vi "记录转表格.vi"(2 "记录":T1(array[cluster])) -> (16 "表格":string[][](array[string]))   [LabVIEW 2019, in "MainPage.lvlib" / "MainPage.lvclass"]
uses:
  MainPage.lvclass
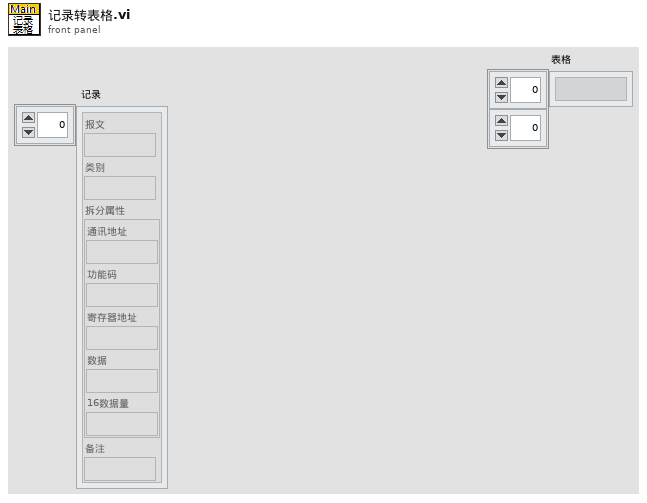
[diagram p1: front panel]
types:
  T1 = cluster{"报文":string, "类别":string, "拆分属性":cluster{"通讯地址":string, "功能码":string, "寄存器地址":string, "数据":string, "16数据量":string}, "备注":string}[]
  T2 = cluster{"报文":string, "类别":string, "拆分属性":cluster{"通讯地址":string, "功能码":string, "寄存器地址":string, "数据":string, "16数据量":string}, "备注":string}
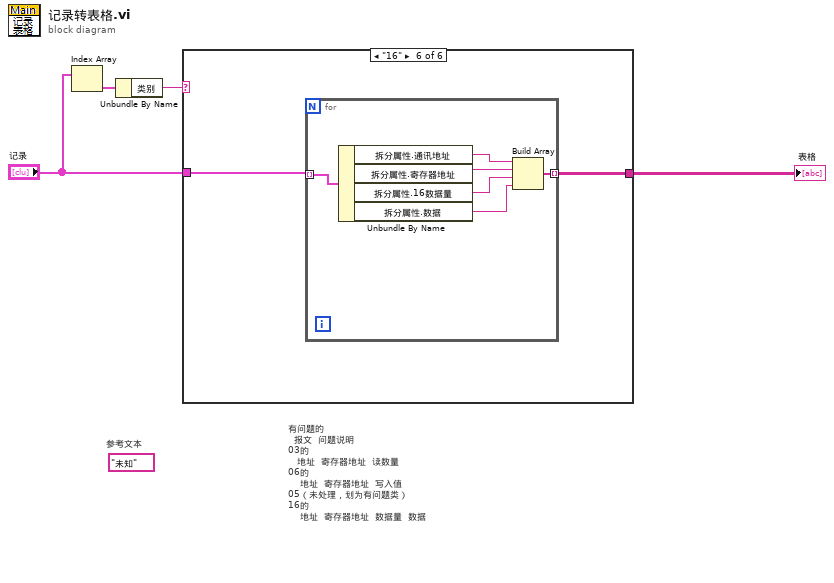
[diagram p0: block diagram]
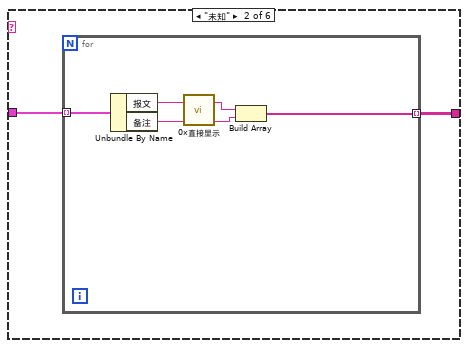
[diagram p3: hidden frame]
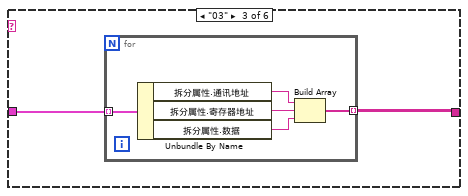
[diagram p4: hidden frame]
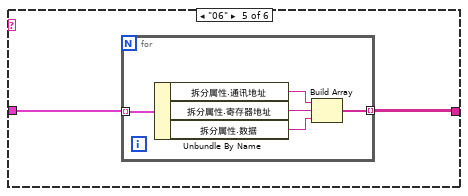
[diagram p6: hidden frame]
diagram:
  (unwired) "未知" ("类别")
  # "参考文本"
  # "有问题的\n  报文  问题说明\n03的\n   地址  寄存器地址  读数量\n06的\n    地址  寄存器地址  写入值\n05（未处理，划为有问题类）\n16的\n    地址  寄存器地址  数据量  数据"
  n1 = Index Array(array="记录") -> (element=w4:T2)  [unwired: 1 in]
  n2 = Unbundle By Name(w4) -> ("类别"=w3:string)
  n3 = case shown="\"16\"" w3 {
    tunnel: "记录" -> [_ w6 w13 _ w20 w27]
    tunnel: [_ w5 w12 _ w19 w26] -> w1
    frame Default {
    }
    frame "未知" {
      n4 = for {
        tunnel: w6 -> [w11] mode=indexing
        tunnel: [w7] -> w5 mode=indexing
        n5 = Unbundle By Name(w11) -> ("报文"=w10:string, "备注"=w8:string)
        n6 = call "0x直接显示.vi"("普通字符串"=w10) -> ("0x普通字符串"=w9:string)  [unwired: 18 in]
        n7 = Build Array(w9, w8) -> (w7:string[])
      }
    }
    frame "03" {
      n8 = for {
        tunnel: w13 -> [w18] mode=indexing
        tunnel: [w14] -> w12 mode=indexing
        n9 = Unbundle By Name(w18) -> ("拆分属性.通讯地址"=w17:string, "拆分属性.寄存器地址"=w16:string, "拆分属性.数据"=w15:string)
        n10 = Build Array(w17, w16, w15) -> (w14:string[])
      }
    }
    frame "05" {
    }
    frame "06" {
      n11 = for {
        tunnel: w20 -> [w25] mode=indexing
        tunnel: [w21] -> w19 mode=indexing
        n12 = Unbundle By Name(w25) -> ("拆分属性.通讯地址"=w24:string, "拆分属性.寄存器地址"=w23:string, "拆分属性.数据"=w22:string)
        n13 = Build Array(w24, w23, w22) -> (w21:string[])
      }
    }
    frame "16" {
      n14 = for {
        tunnel: w27 -> [w33] mode=indexing
        tunnel: [w29] -> w26 mode=indexing
        n15 = Unbundle By Name(w33) -> ("拆分属性.通讯地址"=w32:string, "拆分属性.寄存器地址"=w31:string, "拆分属性.16数据量"=w30:string, "拆分属性.数据"=w28:string)
        n16 = Build Array(w32, w31, w30, w28) -> (w29:string[])
      }
    }
  }
  "表格" <- w1
